vi "test saving tiff stack.vi"() -> ()   [LabVIEW 2018]
panel:
  in  "stop":bool
  out "time for save":dbl
  out "time for process":dbl
  in  "ImageDescriptions":string[](array[string])
  out "error out":errorcluster
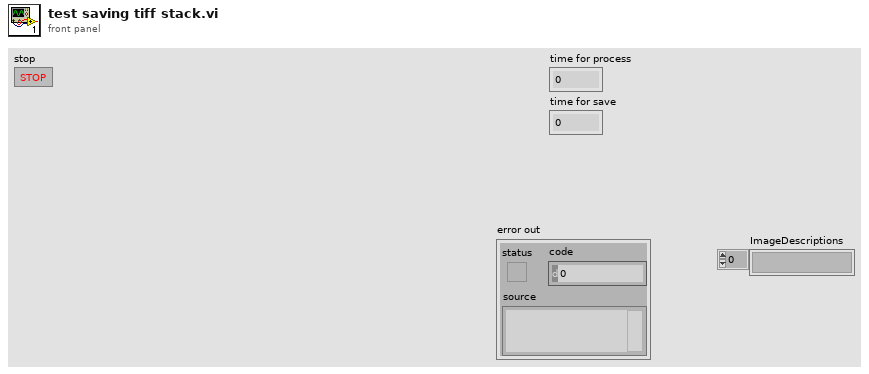
[diagram p1: front panel]
types:
  T1 = typedef "Image Type" = u32
  T2 = typedef "IMAQ Image.ctl" = refnum<image>
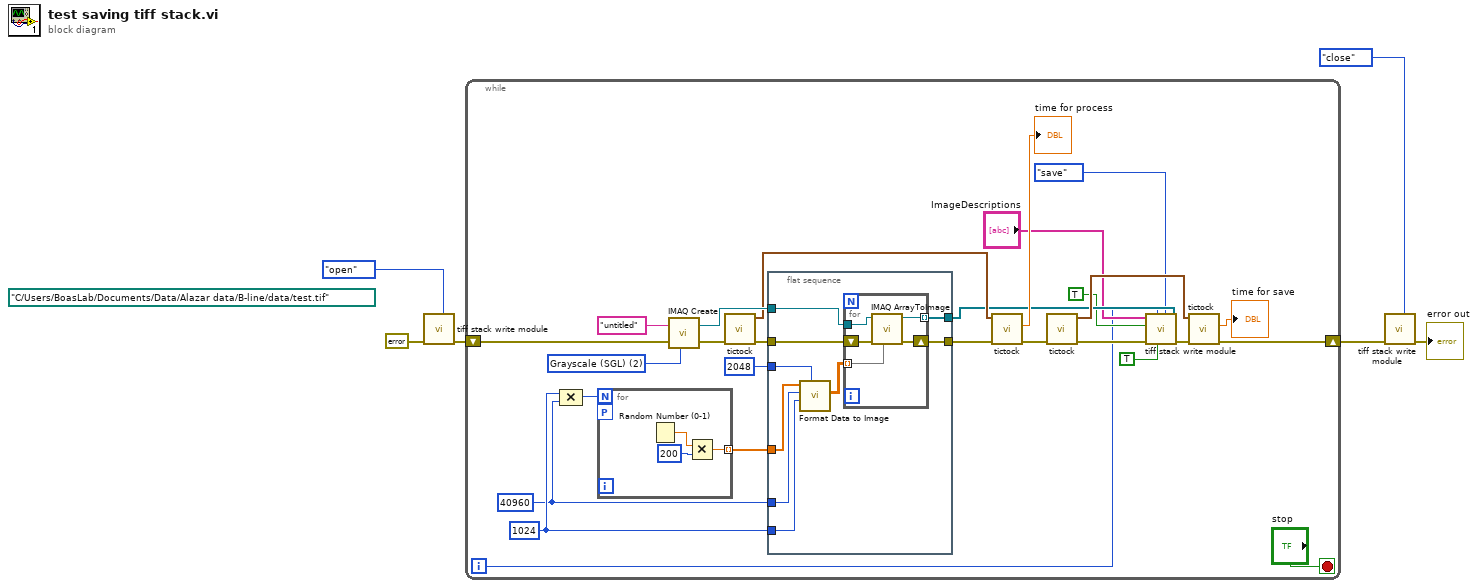
[diagram p0: block diagram]
diagram:
  (unwired) path "C:/Users/BoasLab/Documents/Data/Alazar data/B-line/data/test.tif" ("Path")
  n1 = call "tiff stack write module.vi"("action"=enum16{"open", "save", "close"}."open", "error in"=errorcluster {"status"=FALSE, "code"=0, "source"=""} ("error in (no error)")) -> ("error out"=w5:errorcluster)  [unwired: 9 in]
  n2 = while {
    shift-right: [w10] -> w3
    shift-left: w5 -> [w17]
    i -> [w7]
    stop <- "stop" stop-if-true
    w30 = T1 2 items=["Grayscale (U8)", "Grayscale (I16)", "Grayscale (SGL)", "Complex (CSG)", "RGB (U32)", "HSL (U32)", "RGB (U64)", "Grayscale (U16)"] ("Image Type")
    w20 = 40960
    w21 = 1024
    n3 = Compound Arithmetic op=MULTIPLY(w21, w20) -> (w33:i32)
    n4 = for {
      N: w33 -> [_]
      workers-P: _ -> [_]
      tunnel: [w48] -> w19 mode=indexing
      n5 = Random Number (0-1)() -> (number: 0 to 1=w50:dbl)
      n6 = Multiply(x=w50, y=200) -> (x*y=w48:dbl)
    }
    n7 = call "IMAQ Create"("Image Name"="untitled", "Image Type"=w30, "error in (no error)"=w17) -> ("New Image"=w31:T2, "error out"=w24:errorcluster)  [unwired: 2 in]
    n8 = call "tictock.vi"("error in (no error)"=w24) -> ("error out"=w18:errorcluster, "seconds since 1Jan1904"=w23:timestamp)  [unwired: 8 in, 1 out]
    n9 = flat-sequence {
      tunnel: w31 -> [w42]
      tunnel: [w41] -> w16
      tunnel: [w40] -> w29
      tunnel: 2048 -> [w39]
      tunnel: w21 -> [w38]
      tunnel: w20 -> [w37]
      tunnel: w19 -> [w36]
      tunnel: w18 -> [w34]
      frame #0 {
        n10 = call "Format Data to Image.vi"("#A-lines per B-line"=w39, "Z pixels"=w38, "# B-lines"=w37, "data in"=w36) -> ("float data"=w35:sgl[][][])  [unwired: 6 in, 1 out]
        n11 = for {
          tunnel: w35 -> [w43] mode=indexing
          shift-right: [w46] -> w40
          shift-left: w34 -> [w47]
          tunnel: [w45] -> w41 mode=indexing
          tunnel: w42 -> [w44]
          n12 = call "IMAQ ArrayToImage"("Image Pixels (Float)"=w43, "error in (no error)"=w47, "Image"=w44) -> ("error out"=w46:errorcluster, "Image Out"=w45:T2)  [unwired: 7 in]
        }
      }
    }
    n13 = call "tictock.vi"("error in (no error)"=w29, "seconds since 1Jan1904 2"=w23) -> ("error out"=w28:errorcluster, "Numeric"=→"time for process":dbl)  [unwired: 7 in, 1 out]
    n14 = call "tictock.vi"("error in (no error)"=w28) -> ("error out"=w13:errorcluster, "seconds since 1Jan1904"=w26:timestamp)  [unwired: 8 in, 1 out]
    n15 = call "tiff stack write module.vi"("Array of Images (U8, U16, I16)"=w16, "action"=enum16{"open", "save", "close"}."save", "Add metadata? (T)"=TRUE, "i"=w7, "error in"=w13, "Convert to U16?"=TRUE, "ImageDescriptions"="ImageDescriptions") -> ("error out"=w11:errorcluster)  [unwired: 4 in]
    n16 = call "tictock.vi"("error in (no error)"=w11, "seconds since 1Jan1904 2"=w26) -> ("error out"=w10:errorcluster, "Numeric"=→"time for save":dbl)  [unwired: 7 in, 1 out]
  }
  n17 = call "tiff stack write module.vi"("action"=enum16{"open", "save", "close"}."close", "error in"=w3) -> ("error out"=→"error out":errorcluster)  [unwired: 9 in]
